vi "Read Type ID.vi"(8 "error in (no error)":errorcluster, 11 "ADAS PE Template Controller in":refnum<class "PE Controller.lvclass">) -> (0 "error out":errorcluster, 2 "Type ID":string, 3 "ADAS PE Template Controller out":refnum<class "PE Controller.lvclass">)   [LabVIEW 2020, in "ADAS PE Template.lvlib" / "PE Controller.lvclass"]
uses:
  PE Controller.lvclass
panel:
  # "#via_ignore"
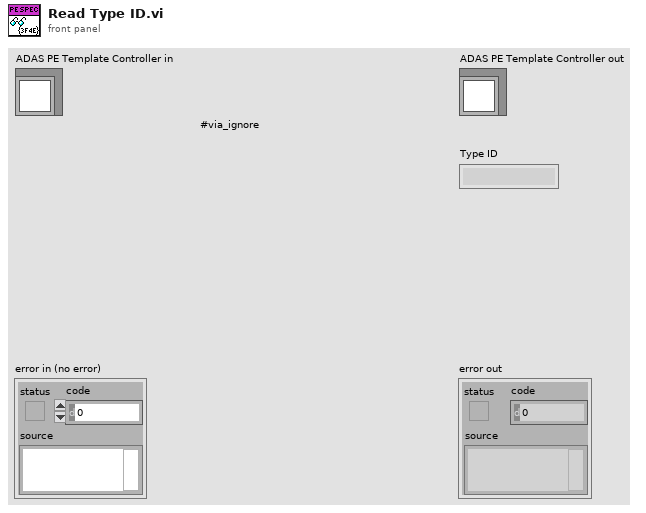
[diagram p1: front panel]
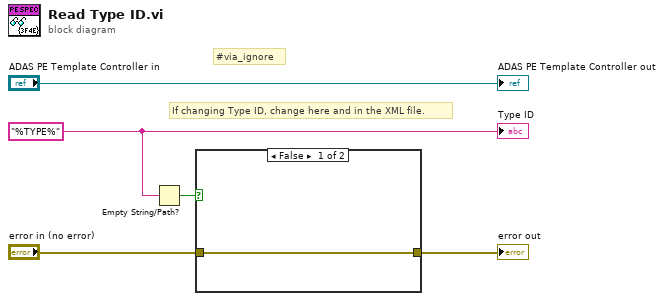
[diagram p0: block diagram]
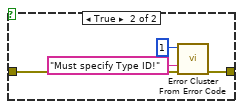
[diagram p2: hidden frame]
diagram:
  w2 = "%TYPE%" ("Unique GUID Constant")
  # "#via_ignore"
  # "If changing Type ID, change here and in the XML file."
  n1 = Empty String/Path?(string/path=w2) -> (empty?=w1:bool)
  n2 = case shown="False" w1 {
    tunnel: "error in (no error)" -> [w6 w10]
    tunnel: [w6 w9] -> w4
    frame False {
    }
    frame True {
      n3 = call <vilib>:"Error Cluster From Error Code.vi"("error in (no error)"=w10, "error message (\"\")"="Must specify Type ID!" ("error message (\"\")"), "error code (0)"=1) -> ("error out"=w9:errorcluster)  [unwired: 6 in]
    }
  }
  "error out" <- w4
  "ADAS PE Template Controller out" <- "ADAS PE Template Controller in"
  "Type ID" <- w2
